vi "Write String.vi"(8 "error in (no error)":errorcluster, 10 "Abs_String.lvclass":refnum<class "Abs_String.lvclass">, 11 "Subset_STR in":refnum<class "Subset_STR.lvclass">) -> (0 "error out":errorcluster, 3 "Subset_STR out":refnum<class "Subset_STR.lvclass">)   [LabVIEW 2021, in "Subset_STR.lvclass"]
uses:
  Subset_STR.lvclass
  Abs_Types/String/Abs_String.lvclass
  Subset_STR.lvclass/Subset_STR.ctl
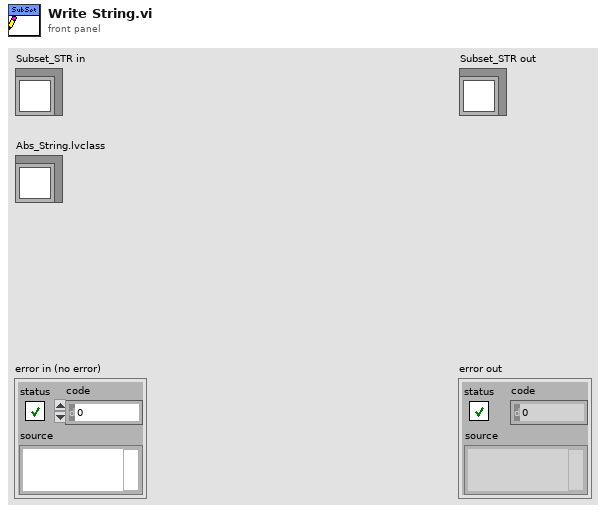
[diagram p1: front panel]
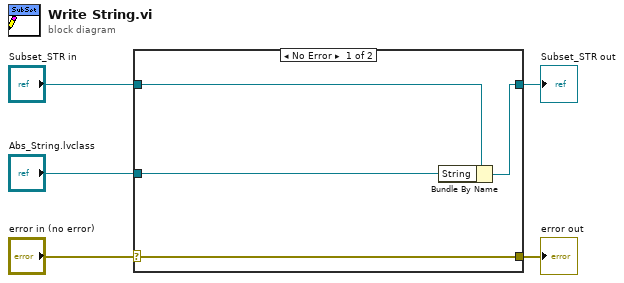
[diagram p0: block diagram]
diagram:
  n1 = case shown="No Error" "error in (no error)" {
    selector: "error in (no error)" -> [w9 w10]
    tunnel: [w9 w10] -> w4
    tunnel: [w7 w11] -> w2
    tunnel: "Subset_STR in" -> [w8 w11]
    tunnel: "Abs_String.lvclass" -> [w6 _]
    frame No Error {
      n2 = Bundle By Name(cluster=w8, "String"=w6) -> (w7:refnum<class "Subset_STR.lvclass">)
    }
    frame Error {
    }
  }
  "error out" <- w4
  "Subset_STR out" <- w2
